vi "VisualizeAppModelValidation.vi"() -> ()   [LabVIEW 2017, in "Visualization.lvlib" / "VisualizeAppModelValidation.lvclass"]
uses:
  VisualizeAppModelValidation.lvclass
  Modules/AppPlugins/ModelValidationPlugin/ModelValidationPlugin.lvclass
  C:/dev/Work/PARTF/Modules/AppPlugins/AppPluginBaseClass/AppPluginsBase.lvclass
  Modules/AppModule/PublicAPI/Arguments/Broadcasts/clStatUpdate.ctl
  VisializeBase_class/Requests/clUserEventType.ctl
  Modules/EventPlugins/EventPluginBaseClass/TypeDefs/clEvtReportArray.ctl
  Modules/EventPlugins/EventPluginBaseClass/TypeDefs/clEvtReport.ctl
  Modules/AppPlugins/AppPluginBaseClass/AppPluginsBase.lvclass/AppPluginsBase.ctl
  Modules/AppPlugins/ModelValidationPlugin/PublicAPI/TypeDef/Output.ctl
  <vilib>/event_ctls.llb/usereventprio.ctl
  Modules/AppPlugins/AppPluginBaseClass/Accessors/Write clEvtReportArray.vi
  <vilib>/Utility/error.llb/Error Cluster From Error Code.vi
  <vilib>/ErrorRing/Error Ring.xnode
  <userlib>/NIST/NISTErrorLib/NISTErrorLib.lvlib
  VisializeBase_class/VisualizeBase_class.lvclass
  Modules/AppModule/AppModule.lvlib
  Modules/EventPlugins/EventPluginBaseClass/EventPluginBaseClass.lvclass
  Modules/PmuImpairModule/PmuImpairModule.lvlib
  Modules/EventModule/EventModule.lvlib
panel:
  out "?":waveform(dbl)(graph)
  out "?":waveform(dbl)(graph)
  out "?":waveform(dbl)(graph)
  in  "btnStop":bool
  out "Status Broadcasts":string
  in  "QueName":string="VisAppQue"
  out "?":waveform(dbl)(graph)
  in  "restart VI":bool
  out "Error Array":errorcluster[][](array[cluster])
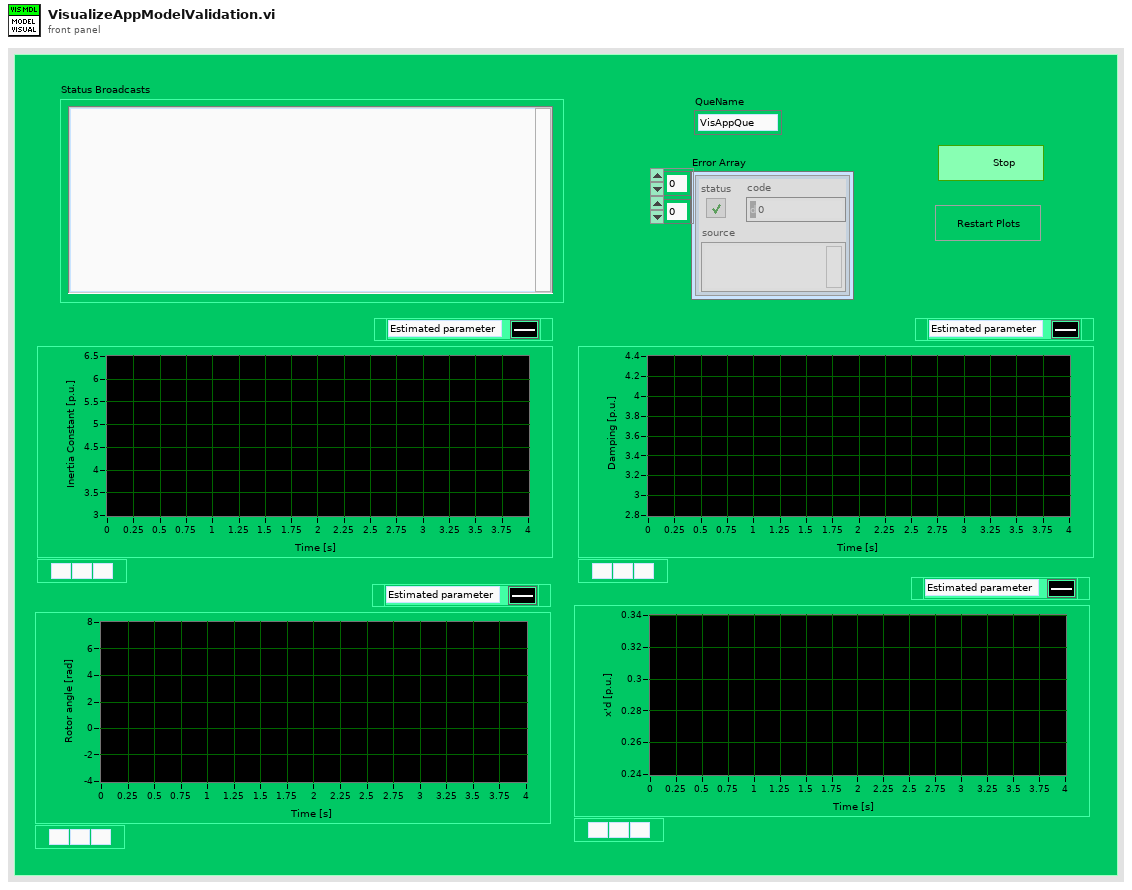
[diagram p1: front panel]
types:
  T1 = typedef "EventPlugins.lvlib/EventPluginBaseClass.lvclass/clEvtReportArray.ctl" = T2[]
  T2 = typedef "EventPlugins.lvlib/EventPluginBaseClass.lvclass/clEvtReport.ctl" = cluster{"Timestamp":dbl, "Synx":cdb[], "Freq":dbl, "ROCOF":dbl, "ID":i16}
  T3 = typedef "AppPlugins.lvlib/ModelValidationPlugin.lvclass/Output.ctl" = cluster{"xk":dbl[][], "Pk":dbl[][], "KalmanGain":dbl[][], "delta_t":dbl}
  T4 = typedef "Visualization.lvlib/VisualizeBase_class.lvclass/clUserEventType.ctl" = cluster{"BusIndex":i8, "Data":variant}
  T5 = typedef "usereventprio.ctl" = enum32{"high priority", "normal priority"}
  T6 = typedef "AppModule.lvlib/clStatUpdate.ctl" = cluster{"Status":string}
  T7 = typedef "Visualization.lvlib/VisualizeBase_class.lvclass/clRequestEvents.ctl" = cluster{"StopRequest":refnum<user-event>}
  T8 = typedef "AppModule.lvlib/clBroadcastEvents.ctl" = cluster{"DidInit":refnum<user-event>, "StatusUpdate":refnum<user-event>, "ErrorReport":refnum<user-event>, "DidStop":refnum<user-event>, "PathToINI":refnum<user-event>, "InputData":refnum<user-event>, "OutputData":refnum<user-event>, "BcAppInfo":refnum<user-event>, "ConfigData":refnum<user-event>}
  T9 = typedef "PmuImpairModule.lvlib/clBroadcastEvents.ctl" = cluster{"DidInit":refnum<user-event>, "StatusUpdate":refnum<user-event>, "ErrorReport":refnum<user-event>, "DidStop":refnum<user-event>, "ImpairConfig":refnum<user-event>, "ImpairParams":refnum<user-event>, "ImpairReports":refnum<user-event>, "PathToPlugin":refnum<user-event>, "BusNumber":refnum<user-event>}
  T10 = typedef "EventModule.lvlib/clBroadcastEvents.ctl" = cluster{"DidInit":refnum<user-event>, "StatusUpdate":refnum<user-event>, "ErrorReport":refnum<user-event>, "DidStop":refnum<user-event>, "ReadEvtConfig":refnum<user-event>, "ReadTimeArray":refnum<user-event>, "ReadEvtParams":refnum<user-event>, "GetEvtReportArray":refnum<user-event>, "ReadPathToPlugin":refnum<user-event>, "GetEvtSignal":refnum<user-event>, "ReadBusNumber":refnum<user-event>}
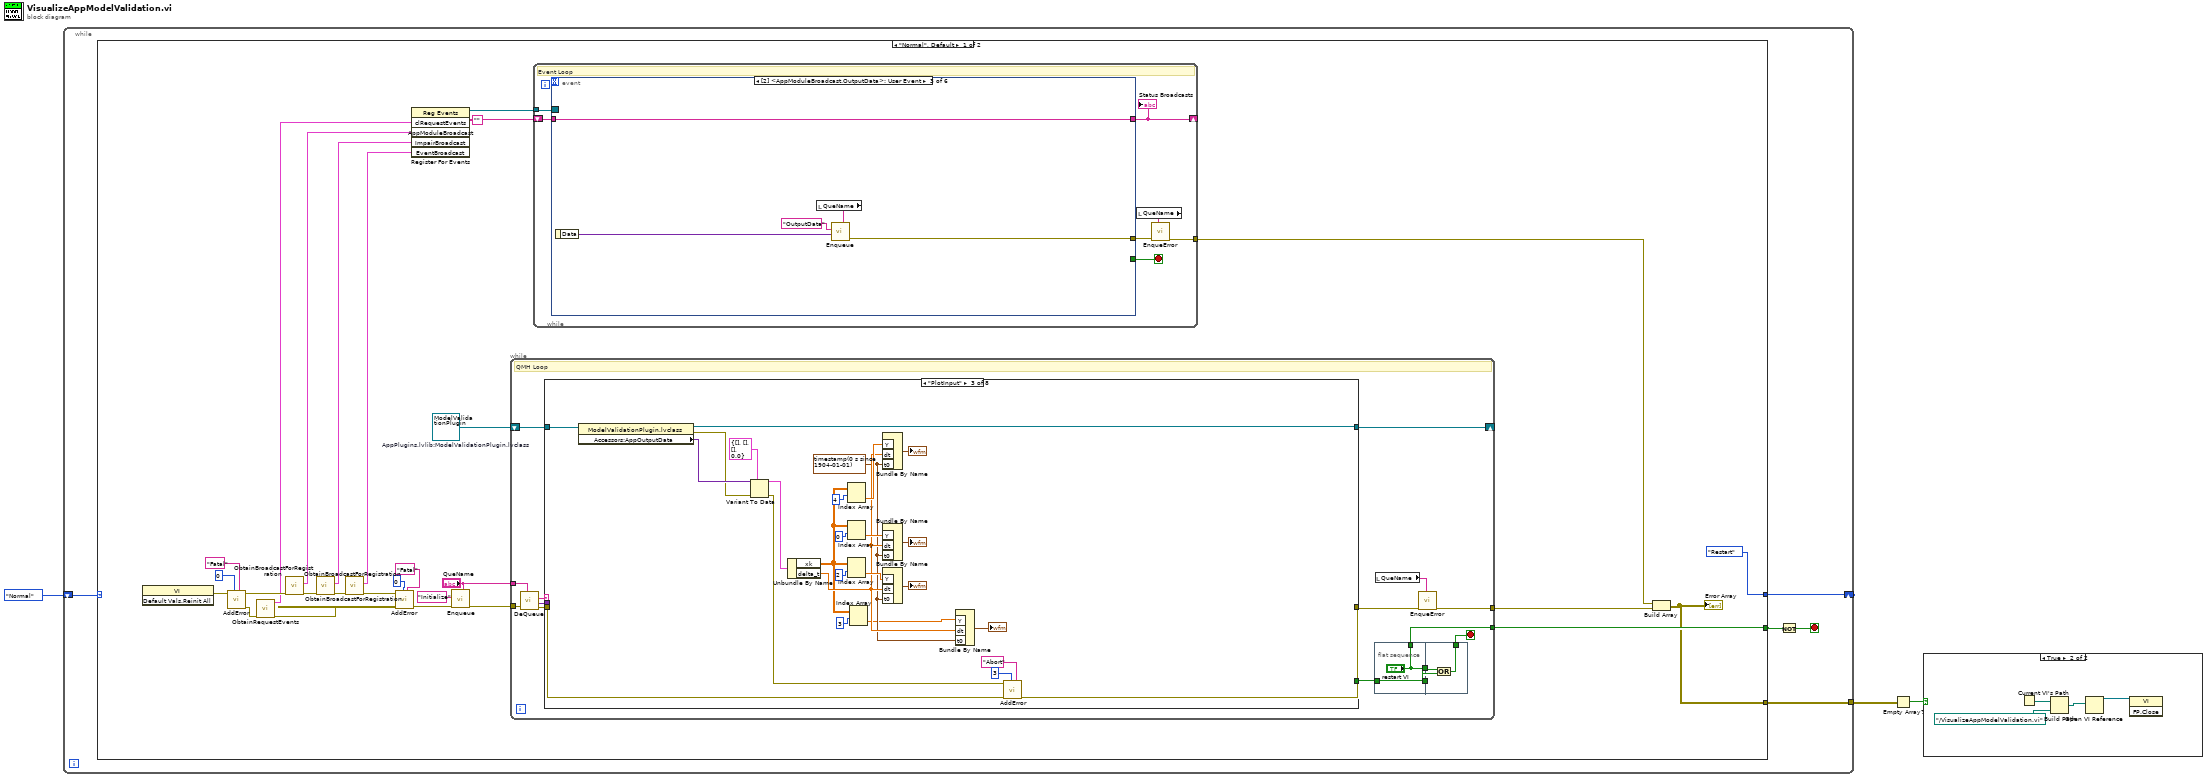
[diagram p0: block diagram]
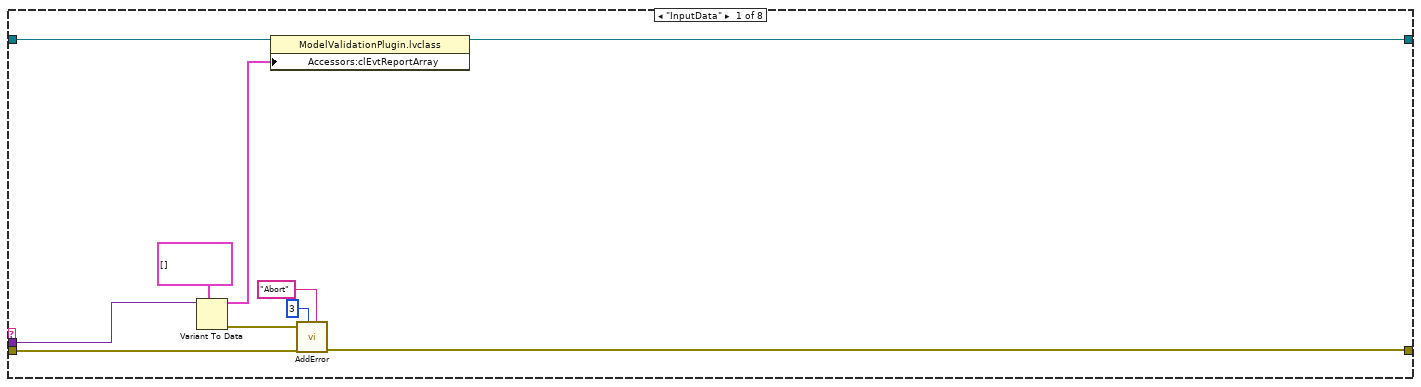
[diagram p3: hidden frame]
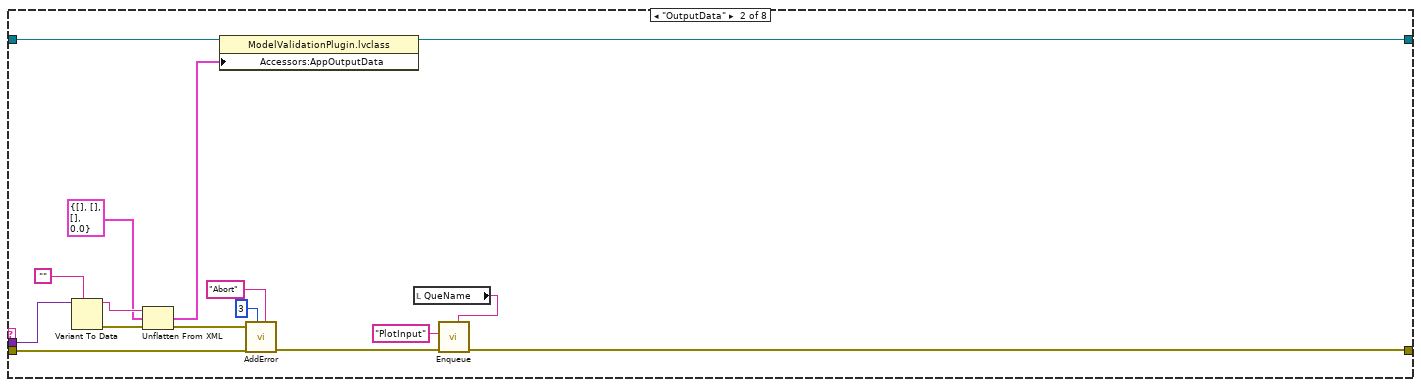
[diagram p4: hidden frame]
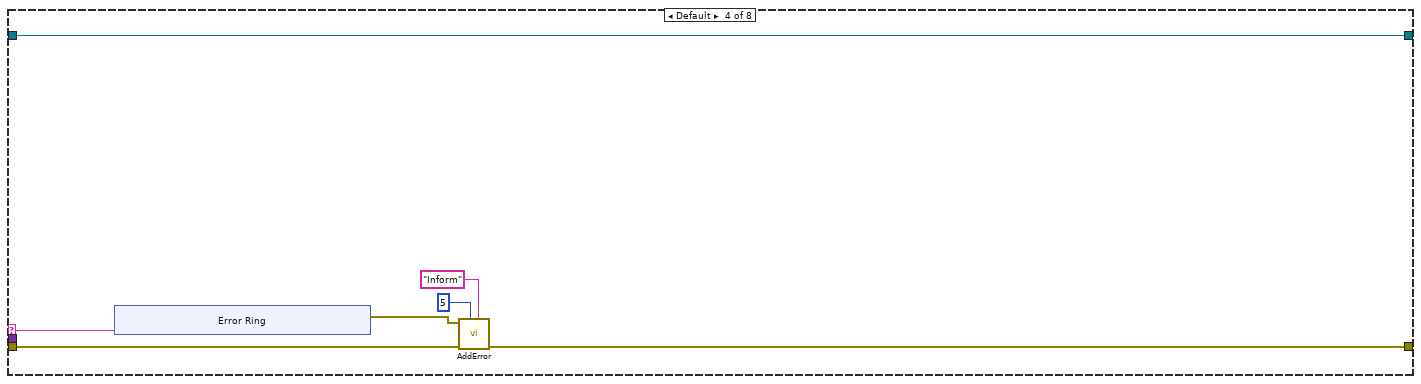
[diagram p5: hidden frame]
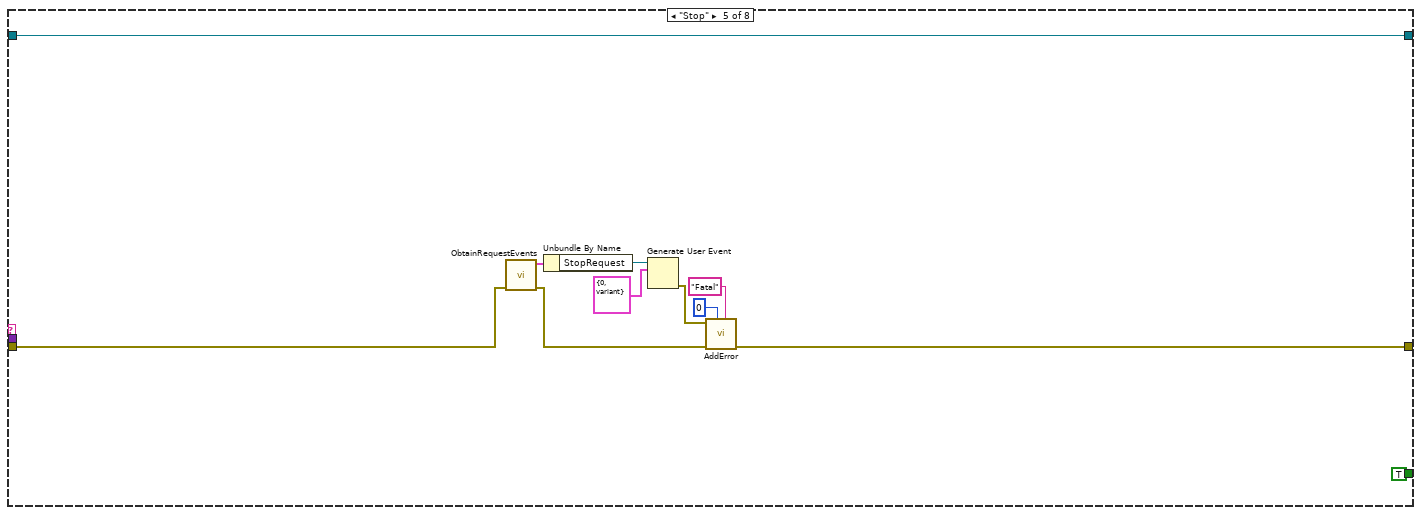
[diagram p6: hidden frame]
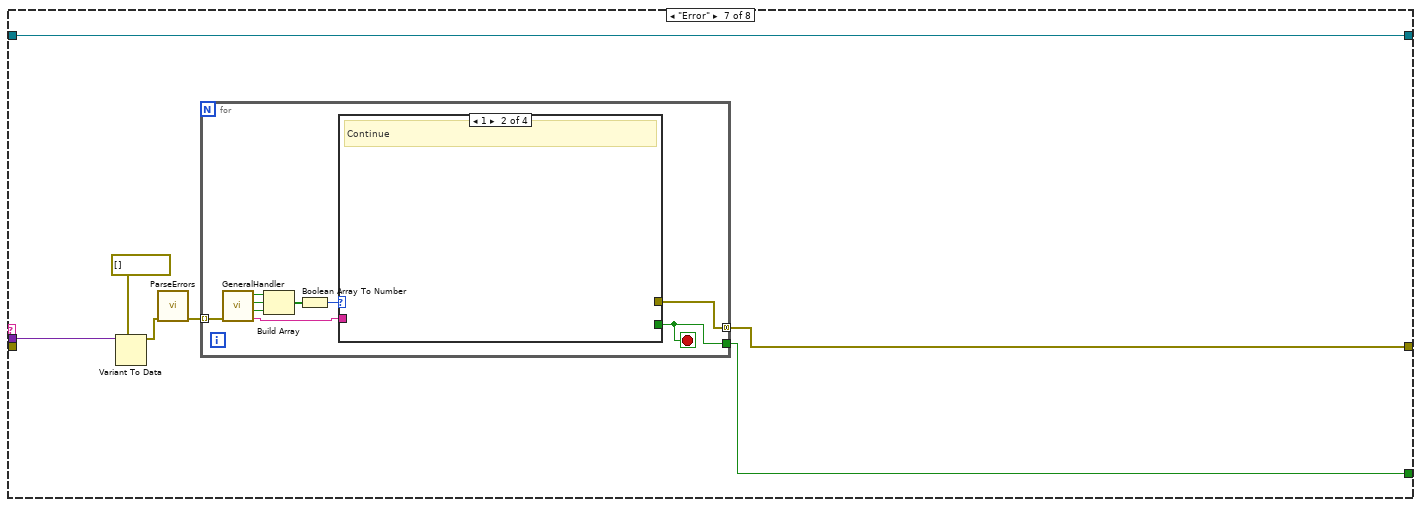
[diagram p8: hidden frame]
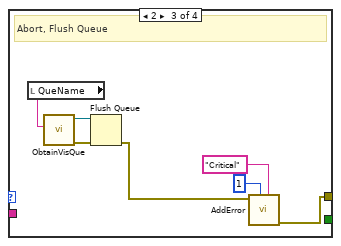
[diagram p10: hidden frame]
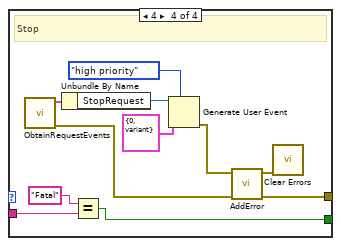
[diagram p11: hidden frame]
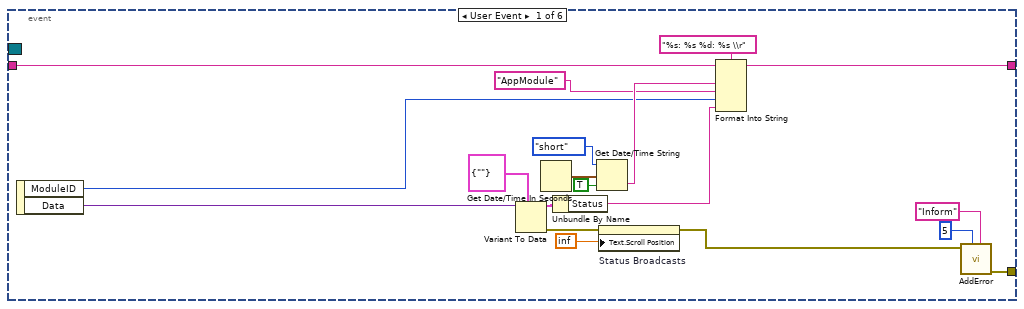
[diagram p13: hidden frame]
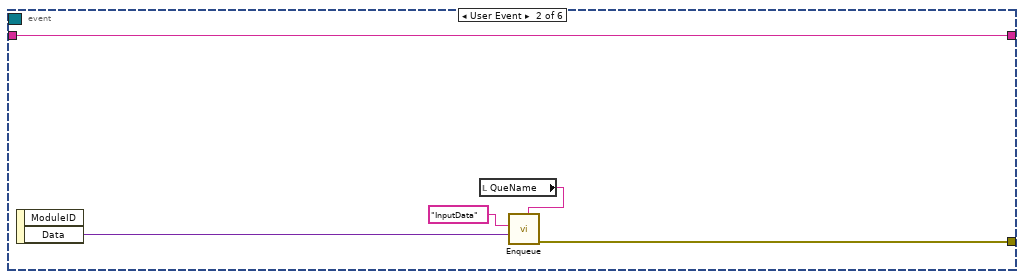
[diagram p14: hidden frame]
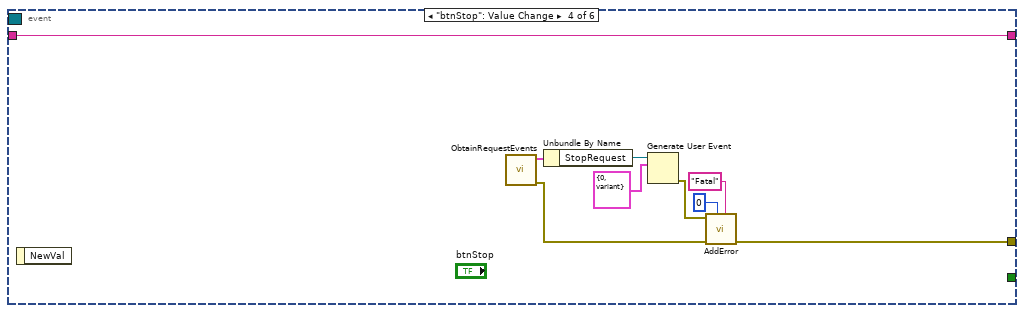
[diagram p15: hidden frame]
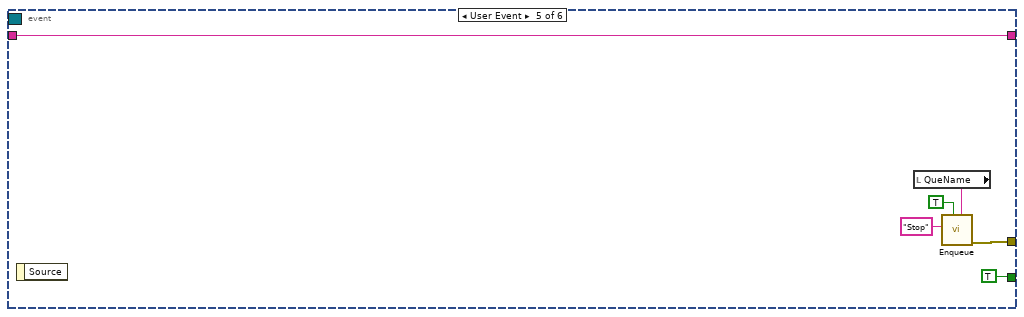
[diagram p16: hidden frame]
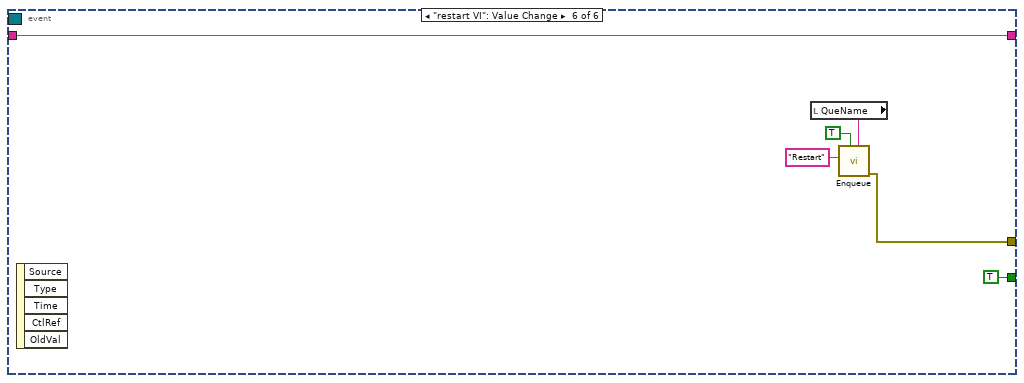
[diagram p17: hidden frame]
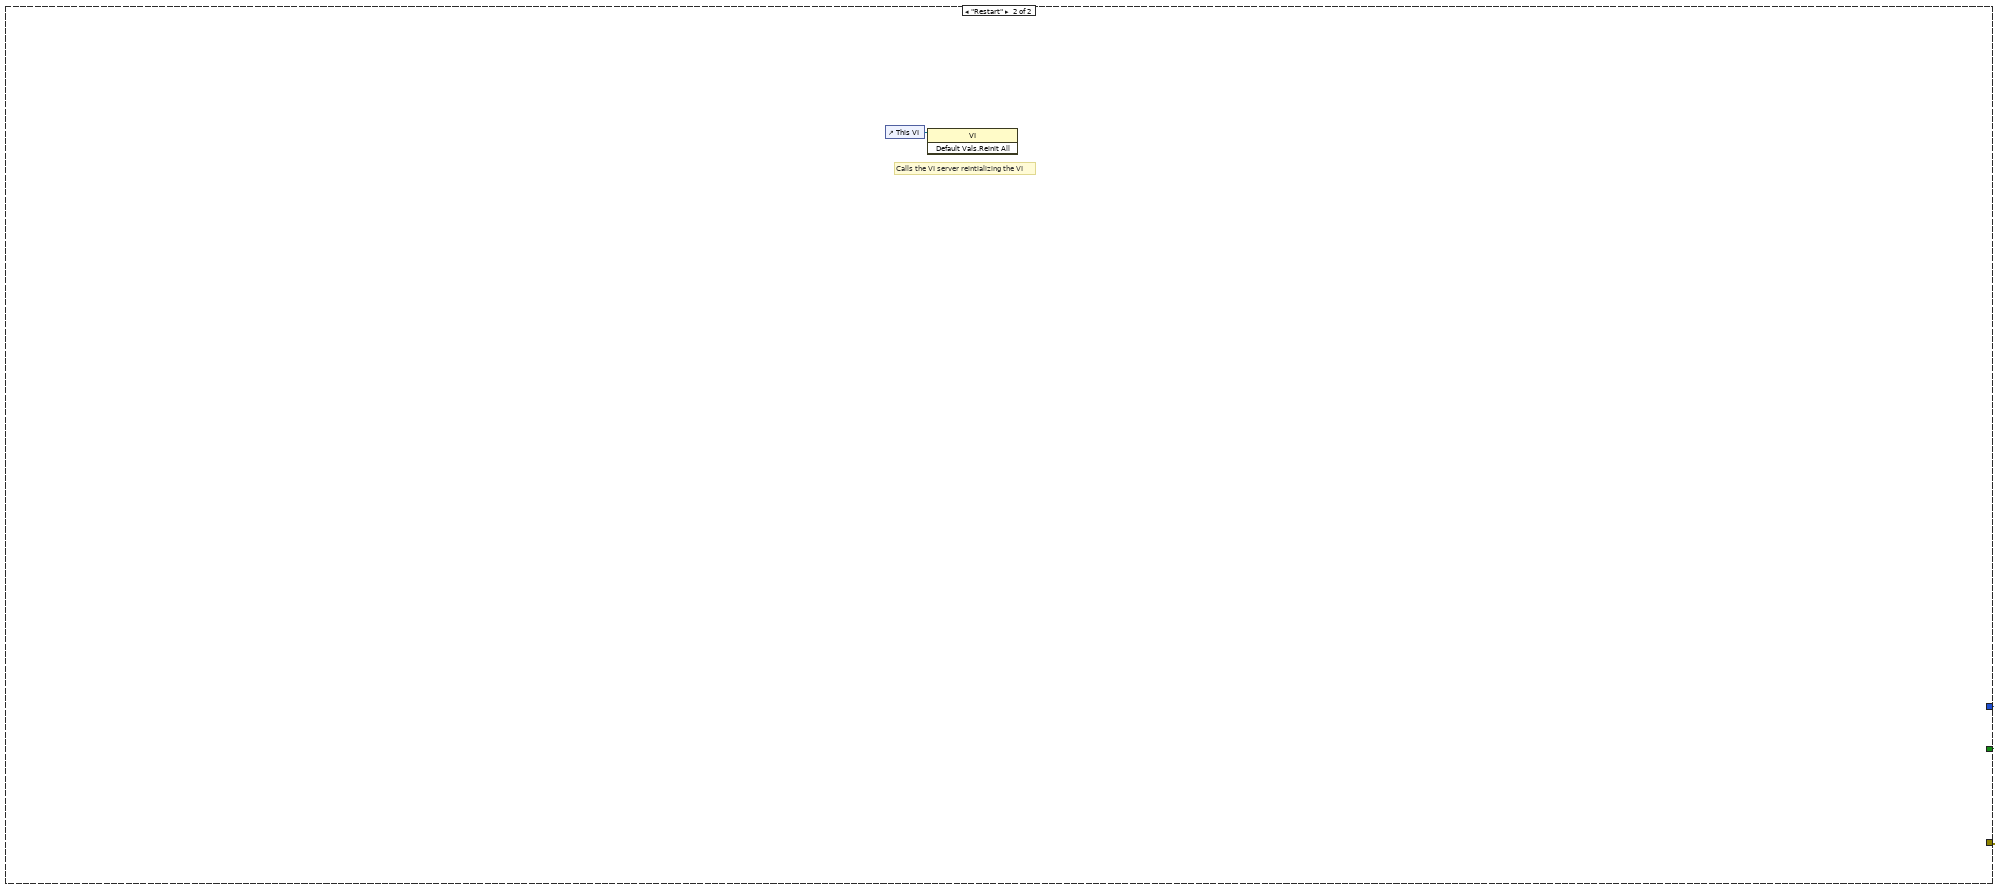
[diagram p18: hidden frame]
diagram:
  n1 = while {
    shift-right: [w5] -> _
    shift-left: enum16{"Normal", "Restart"}."Normal" -> [w6]
    tunnel: [w4] -> w1
    stop <- w7 stop-if-true
    n2 = case shown="\"Normal\", Default" w6 {
      tunnel: [w12 TRUE] -> w8
      tunnel: [enum16{"Normal", "Restart"}."Restart" enum16{"Normal", "Restart"}."Normal"] -> w5
      tunnel: [w10 errorcluster[][] []] -> w4
      frame "Normal", Default {
        w9 = refnum<class "ModelValidationPlugin.lvclass"> refnum  # AppPlugins.lvlib:ModelValidationPlugin.lvclass
        n3 = invoke class="VI" method="Default Vals.Reinit All"() -> (error out=w18:errorcluster)  [unwired: 3 in, 2 out]
        n4 = call <userlib>:"AddError.vi"("Severity"="Fatal", "Priority"=u8 0, "error in (no error)"=w18) -> ("ErrorArray"=w33:errorcluster[], "error out"=w32:errorcluster)  [unwired: 7 in]
        n5 = call "ObtainRequestEvents.vi"("Error"=w33) -> ("Error"=w29:errorcluster[], "clRequestEvents"=w31:T7)  [unwired: 9 in]
        n6 = call "ObtainBroadcastForRegistration.vi"("error in (no error)"=w32) -> ("error out"=w17:errorcluster, "AppModuleBroadcast"=w30:T8)  [unwired: 9 in]
        n7 = call "ObtainBroadcastForRegistration.vi"("error in (no error)"=w17) -> ("error out"=w16:errorcluster, "ImpairBroadcast"=w15:T9)  [unwired: 9 in]
        n8 = call "ObtainBroadcastForRegistration.vi"("error in (no error)"=w16) -> ("error out"=w14:errorcluster, "EventBroadcast"=w13:T10)  [unwired: 9 in]
        n9 = call <userlib>:"AddError.vi"("Severity"="Fatal", "Priority"=u8 0, "ErrorArray"=w29, "error in (no error)"=w14) -> ("ErrorArray"=w27:errorcluster[])  [unwired: 6 in, 1 out]
        n10 = register-events(w31, w30, w15, w13) -> (reference out=w22:refnum<event-registration>)  [unwired: 2 in, 1 out]
        n11 = call "Enqueue.vi"("QueName"="QueName", "Error"=w27, "Message"="Initialize") -> ("Error"=w24:errorcluster[])  [unwired: 8 in]
        n12 = while {
          tunnel: w24 -> [w50]
          tunnel: "QueName" -> [w49]
          tunnel: [w43] -> w21
          shift-right: [w41] -> _
          shift-left: w9 -> [w42]
          tunnel: [w40] -> w12
          stop <- w36 stop-if-true
          # "QMH Loop"
          n13 = call "DeQueue.vi"("QueName"=w49, "Error"=w50) -> ("Error"=w46:errorcluster[], "Data"=w47:variant, "Message"=w48:string)  [unwired: 7 in]
          n14 = case shown="\"PlotInput\"" w48 {
            selector: w48 -> [_ _ _ w114 _ _ _ _]
            tunnel: w47 -> [w63 w79 _ _ _ _ w138 _]
            tunnel: w46 -> [w59 w78 w105 w113 w124 w134 _ w169]
            tunnel: [w58 w74 w104 w109 w125 w134 w140 w169] -> w45
            tunnel: [_ _ _ _ TRUE _ w141 _] -> w38
            tunnel: w42 -> [w65 w81 w107 w108 w122 w133 w135 w170]
            tunnel: [w64 w80 w106 w108 w122 w133 w135 w170] -> w41
            frame "InputData" {
              n15 = Variant To Data(type=T1 [] ("clEvtReportArray"), Variant=w63) -> (data=w61:T1, error out=w60:errorcluster)  [unwired: 1 in]
              n16 = property class="ModelValidationPlugin.lvclass"(reference=w65, "Accessors:clEvtReportArray"=w61) -> (reference out=w64:refnum<class "ModelValidationPlugin.lvclass">)  [unwired: 1 in, 1 out]
              n17 = call <userlib>:"AddError.vi"("Severity"="Abort", "Priority"=u8 3, "ErrorArray"=w59, "error in (no error)"=w60) -> ("ErrorArray"=w58:errorcluster[])  [unwired: 6 in, 1 out]
            }
            frame "OutputData" {
              n18 = Variant To Data(type="", Variant=w79) -> (data=w71:string, error out=w69:errorcluster)  [unwired: 1 in]
              n19 = Unflatten From XML(xml string=w71, type=T3 {"xk"=[], "Pk"=[], "KalmanGain"=[], "delta_t"=0.0} ("ModelValidationOutput"), error in (no error)=w69) -> (value=w67:T3, error out=w68:errorcluster)
              n20 = property class="ModelValidationPlugin.lvclass"(reference=w81, "Accessors:AppOutputData"=w67) -> (reference out=w80:refnum<class "ModelValidationPlugin.lvclass">)  [unwired: 1 in, 1 out]
              n21 = call <userlib>:"AddError.vi"("Severity"="Abort", "Priority"=u8 3, "ErrorArray"=w78, "error in (no error)"=w68) -> ("ErrorArray"=w75:errorcluster[])  [unwired: 6 in, 1 out]
              n22 = local read "QueName"() -> (w72:string)
              n23 = call "Enqueue.vi"("QueName"=w72, "Error"=w75, "Message"="PlotInput") -> ("Error"=w74:errorcluster[])  [unwired: 8 in]
            }
            frame "PlotInput" {
              w89 = timestamp(0 s since 1904-01-01) ("t0")
              n24 = property class="ModelValidationPlugin.lvclass"(reference=w107) -> (reference out=w106:refnum<class "ModelValidationPlugin.lvclass">, error out=w100:errorcluster, "Accessors:AppOutputData"=w101:variant)  [unwired: 1 in]
              n25 = Variant To Data(error in=w100, type=T3 {"xk"=[], "Pk"=[], "KalmanGain"=[], "delta_t"=0.0} ("ModelValidationOutput"), Variant=w101) -> (data=w98:T3, error out=w96:errorcluster)
              n26 = Unbundle By Name(w98) -> ("xk"=w87:dbl[][], "delta_t"=w90:dbl)
              n27 = Index Array(array=w87, index (row)=4 ("disabled index (col)")) -> (element=w94:dbl[])  [unwired: 1 in]
              n28 = Index Array(array=w87, index (row)=0 ("disabled index (col)")) -> (element=w92:dbl[])  [unwired: 1 in]
              n29 = Index Array(array=w87, index (row)=2 ("disabled index (col)")) -> (element=w97:dbl[])  [unwired: 1 in]
              n30 = Index Array(array=w87, index (row)=3 ("index (col)")) -> (element=w86:dbl[])  [unwired: 1 in]
              n31 = Bundle By Name("Y"=w94, "dt"=w90, "t0"=w89) -> (→"?":waveform(dbl))  [unwired: 1 in]
              n32 = Bundle By Name("Y"=w92, "dt"=w90, "t0"=w89) -> (→"?":waveform(dbl))  [unwired: 1 in]
              n33 = Bundle By Name("Y"=w97, "dt"=w90, "t0"=w89) -> (→"?":waveform(dbl))  [unwired: 1 in]
              n34 = Bundle By Name("Y"=w86, "dt"=w90, "t0"=w89) -> (→"?":waveform(dbl))  [unwired: 1 in]
              n35 = call <userlib>:"AddError.vi"("Severity"="Abort", "Priority"=u8 3, "ErrorArray"=w105, "error in (no error)"=w96) -> ("ErrorArray"=w104:errorcluster[])  [unwired: 6 in, 1 out]
            }
            frame Default {
              n36 = xnode "Error Ring"("parameter 0"=w114) -> ("error out"=w112:errorcluster)
              n37 = call <userlib>:"AddError.vi"("Severity"="Inform", "Priority"=u8 5, "ErrorArray"=w113, "error in (no error)"=w112) -> ("ErrorArray"=w109:errorcluster[])  [unwired: 6 in, 1 out]
            }
            frame "Stop" {
              n38 = call "ObtainRequestEvents.vi"("Error"=w124) -> ("Error"=w123:errorcluster[], "clRequestEvents"=w126:T7)  [unwired: 9 in]
              n39 = Unbundle By Name(w126) -> ("StopRequest"=w127:refnum<user-event>)
              n40 = Generate User Event(user event=w127, event data cluster=T4 {"BusIndex"=0, "Data"=variant} ("clEventType")) -> (error out=w129:errorcluster)  [unwired: 2 in, 1 out]
              n41 = call <userlib>:"AddError.vi"("Severity"="Fatal", "Priority"=u8 0, "ErrorArray"=w123, "error in (no error)"=w129) -> ("ErrorArray"=w125:errorcluster[])  [unwired: 6 in, 1 out]
            }
            frame "Initialize" {
            }
            frame "Error" {
              n42 = Variant To Data(type=errorcluster[] [], Variant=w138) -> (data=w136:errorcluster[])  [unwired: 1 in, 1 out]
              n43 = call <userlib>:"ParseErrors.vi"("ErrorArray"=w136) -> ("ErrorArray"=w139:errorcluster[])  [unwired: 8 in, 2 out]
              n44 = for {
                tunnel: w139 -> [w150] mode=indexing
                tunnel: [w144] -> w140 mode=concatenating
                tunnel: [w142] -> w141
                stop <- w142 stop-if-true
                n45 = call <userlib>:"GeneralHandler.vi"("error in (no error)"=w150) -> ("Severity"=w143:string, "Stop"=w147:bool, "Abort"=w148:bool, "Continue"=w149:bool)  [unwired: 7 in]
                n46 = Build Array(w149, w148, w147) -> (w146:bool[])
                n47 = Boolean Array To Number(Boolean array=w146) -> (number=w145:u32)
                n48 = case shown="1" w145 {
                  tunnel: [_ _ w155 w166] -> w144
                  tunnel: w143 -> [_ _ _ w160]
                  tunnel: [_ _ _ w158] -> w142
                  frame 0, Default {
                    # "No Dialog"
                  }
                  frame 1 {
                    # "Continue"
                  }
                  frame 2 {
                    # "Abort, Flush Queue"
                    n49 = local read "QueName"() -> (w151:string)
                    n50 = call "ObtainVisQue.vi"("QueName"=w151) -> ("error out"=w157:errorcluster, "queue out"=w156:refnum<queue>)  [unwired: 9 in]
                    n51 = Flush Queue(queue=w156, error in (no error)=w157) -> (error out=w154:errorcluster)  [unwired: 2 out]
                    n52 = call <userlib>:"AddError.vi"("Severity"="Critical" ("String"), "Priority"=u8 1, "error in (no error)"=w154) -> ("ErrorArray"=w155:errorcluster[])  [unwired: 7 in, 1 out]
                  }
                  frame 4 {
                    # "Stop"
                    n53 = call "ObtainRequestEvents.vi"() -> ("Error"=w164:errorcluster[], "clRequestEvents"=w168:T7)  [unwired: 10 in]
                    n54 = Unbundle By Name(w168) -> ("StopRequest"=w167:refnum<user-event>)
                    n55 = Equal?(x="Fatal", y=w160) -> (x = y?=w158:bool)
                    n56 = Generate User Event(priority (normal)=usereventprio."high priority", user event=w167, event data cluster=T4 {"BusIndex"=0, "Data"=variant} ("event data")) -> (error out=w165:errorcluster)  [unwired: 1 in, 1 out]
                    n57 = call <userlib>:"AddError.vi"("ErrorArray"=w164, "error in (no error)"=w165) -> ("ErrorArray"=w166:errorcluster[], "error out"=w161:errorcluster)  [unwired: 8 in]
                    n58 = call <vilib>:"Clear Errors.vi"("error in (no error)"=w161) -> ()  [unwired: 5 in, 2 out]
                  }
                }
              }
            }
            frame "Restart" {
            }
          }
          n59 = flat-sequence {
            tunnel: ["restart VI"] -> w40
            tunnel: ["restart VI"] -> w39
            tunnel: w38 -> [w51]
            tunnel: [w51] -> w37
            tunnel: w39 -> [w55]
            tunnel: w37 -> [w54]
            tunnel: [w53] -> w36
            frame #0 {
            }
            frame #1 {
              n60 = Or(x=w54, y=w55) -> (x .or. y?=w53:bool)
            }
          }
          n61 = local read "QueName"() -> (w44:string)
          n62 = call "EnqueError.vi"("QueName"=w44, "Error"=w45) -> ("Error"=w43:errorcluster[])  [unwired: 9 in]
        }
        n63 = while {
          tunnel: [w176] -> w20
          tunnel: w22 -> [w174]
          shift-right: [w171] -> _
          shift-left: "" -> [w172]
          stop <- w173 stop-if-true
          # "Event Loop"
          n64 = event shown="[2] <AppModuleBroadcast.OutputData>: User Event" {
            selector: w174 -> [_ _ _ _ _ _]
            dyn-events: _ -> [_ _ _ _ _ _]
            timeout: _ -> [_ _ _ _ _ _]
            tunnel: [w185 w200 w205 w210 w218 w222] -> w177
            tunnel: [_ _ _ _ TRUE TRUE] -> w173
            tunnel: w172 -> [w196 w198 w202 w207 w216 w227]
            tunnel: [w189 w198 w202 w207 w216 w227] -> w171
            event User Event {
              n65 = event-data() -> ("ModuleID"=w179:i32, "Data"=w195:variant)  [unwired: 1 in]
              n66 = Variant To Data(type=T6 {"Status"=""} ("clStatUpdate"), Variant=w195) -> (data=w193:T6, error out=w186:errorcluster)  [unwired: 1 in]
              n67 = Get Date/Time In Seconds() -> (seconds since 1Jan1904=w190:timestamp)
              n68 = Unbundle By Name(w193) -> ("Status"=w180:string)
              n69 = Get Date/Time String(date format (0)=enum16{"short", "long", "abbreviated"}."short", seconds (now)=w190, want seconds? (F)=TRUE) -> (time string=w187:string)  [unwired: 1 out]
              n70 = property on="Status Broadcasts" class="Str"(error in=w186, "Text.Scroll Position"=inf) -> (error out=w184:errorcluster)  [unwired: 1 in, 1 out]
              n71 = Format Into String(format string="%s: %s %d: %s \\r", initial string=w196, w187, "AppModule", w179, w180) -> (resulting string=w189:string)  [unwired: 1 in, 1 out]
              n72 = call <userlib>:"AddError.vi"("Severity"="Inform", "Priority"=u8 5, "error in (no error)"=w184) -> ("ErrorArray"=w185:errorcluster[])  [unwired: 7 in, 1 out]
            }
            event User Event {
              n73 = event-data() -> ("Data"=w201:variant)  [unwired: 1 in, 1 out]
              n74 = local read "QueName"() -> (w197:string)
              n75 = call "Enqueue.vi"("QueName"=w197, "Data"=w201, "Message"="InputData") -> ("Error"=w200:errorcluster[])  [unwired: 8 in]
            }
            event User Event {
              n76 = event-data() -> ("Data"=w206:variant)  [unwired: 1 in]
              n77 = local read "QueName"() -> (w203:string)
              n78 = call "Enqueue.vi"("QueName"=w203, "Data"=w206, "Message"="OutputData") -> ("Error"=w205:errorcluster[])  [unwired: 8 in]
            }
            event "btnStop": Value Change {
              n79 = event-data() -> ()  [unwired: 1 in, 1 out]
              n80 = call "ObtainRequestEvents.vi"() -> ("Error"=w212:errorcluster[], "clRequestEvents"=w215:T7)  [unwired: 10 in]
              n81 = Unbundle By Name(w215) -> ("StopRequest"=w214:refnum<user-event>)
              n82 = Generate User Event(user event=w214, event data cluster=T4 {"BusIndex"=0, "Data"=variant} ("clEventType")) -> (error out=w211:errorcluster)  [unwired: 2 in, 1 out]
              n83 = call <userlib>:"AddError.vi"("Severity"="Fatal", "Priority"=u8 0, "ErrorArray"=w212, "error in (no error)"=w211) -> ("ErrorArray"=w210:errorcluster[])  [unwired: 6 in, 1 out]
            }
            event User Event {
              n84 = event-data() -> ()  [unwired: 1 in, 1 out]
              n85 = local read "QueName"() -> (w220:string)
              n86 = call "Enqueue.vi"("QueName"=w220, "Priority? (F)"=TRUE, "Message"="Stop") -> ("Error"=w218:errorcluster[])  [unwired: 8 in]
            }
            event "restart VI": Value Change {
              n87 = event-data() -> ()  [unwired: 1 in, 5 out]
              n88 = local read "QueName"() -> (w224:string)
              n89 = call "Enqueue.vi"("QueName"=w224, "Priority? (F)"=TRUE, "Message"="Restart") -> ("Error"=w222:errorcluster[])  [unwired: 8 in]
            }
          }
          "Status Broadcasts" <- w171
          n90 = local read "QueName"() -> (w175:string)
          n91 = call "EnqueError.vi"("QueName"=w175, "Error"=w177) -> ("Error"=w176:errorcluster[])  [unwired: 9 in]
        }
        n92 = Build Array(w20, w21) -> (w10:errorcluster[][])
        "Error Array" <- w10
      }
      frame "Restart" {
        # "Calls the VI server reintializing the VI"
        n93 = control-ref of="This VI"() -> (w229:refnum<vi>)
        n94 = invoke class="VI" method="Default Vals.Reinit All"(reference=w229) -> ()  [unwired: 2 in, 3 out]
      }
    }
    n95 = Not(x=w8) -> (.not. x?=w7:bool)
  }
  n96 = Empty Array?(array=w1) -> (empty?=w2:bool)
  n97 = case shown="True" w2 {
    frame False {
    }
    frame True {
      n98 = Current VI's Path() -> (path=w234:path)
      n99 = Build Path(base path=w234, name or relative path=path "../VisualizeAppModelValidation.vi") -> (appended path=w232:path)
      n100 = Open VI Reference(vi path=w232) -> (vi reference=w235:refnum<vi>)  [unwired: 5 in, 1 out]
      n101 = invoke class="VI" method="FP.Close"(reference=w235) -> ()  [unwired: 2 in, 3 out]
    }
  }
